vi "Ramp Sequence.vi"(0 "start":dbl format="%#_13p", 5 "end":dbl format="%#_13p", 7 "delta":dbl format="%#_13p", 11 "error in":errorcluster) -> (4 "Ramp Pattern":dbl[](array[numeric]), 15 "error out":errorcluster)   [LabVIEW 2019]
uses:
  <vilib>/Analysis/1siggen.llb/Ramp Pattern by Delta.vi
  <vilib>/Analysis/NI_AALBase.lvlib
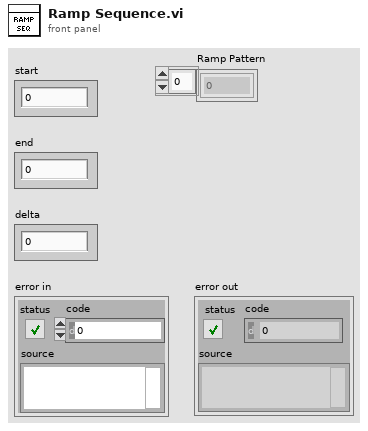
[diagram p1: front panel]
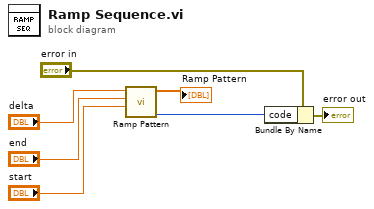
[diagram p0: block diagram]
diagram:
  n1 = call-poly <vilib>:"Ramp Pattern.vi"("start"="start", "end"="end", "delta"="delta") -> ("error"=w4:i32, "Ramp Pattern"=→"Ramp Pattern":dbl[])  [unwired: 6 in, 1 out]
  n2 = Bundle By Name(cluster="error in", "code"=w4) -> (→"error out":errorcluster)
